vi "Graph Closed.vi"(8 "error in (no error)":errorcluster, 10 "Closed Graph":refnum<class "Message Enqueuer.lvclass">, 11 "Mag Lab Measure Base in":refnum<class "Mag Lab Measure Base.lvclass">) -> (0 "error out":errorcluster, 3 "Mag Lab Measure Base out":refnum<class "Mag Lab Measure Base.lvclass">)   [LabVIEW 2015, in "Mag Lab Measure Base.lvclass"]
uses:
  Mag Lab Measure Base.lvclass
  <vilib>/ActorFramework/Message Enqueuer/Message Enqueuer.lvclass
  Mag Lab Measure Base.lvclass/Mag Lab Measure Base.ctl
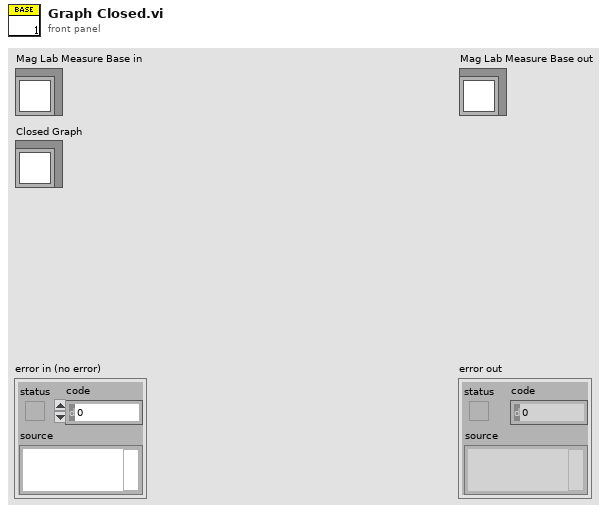
[diagram p1: front panel]
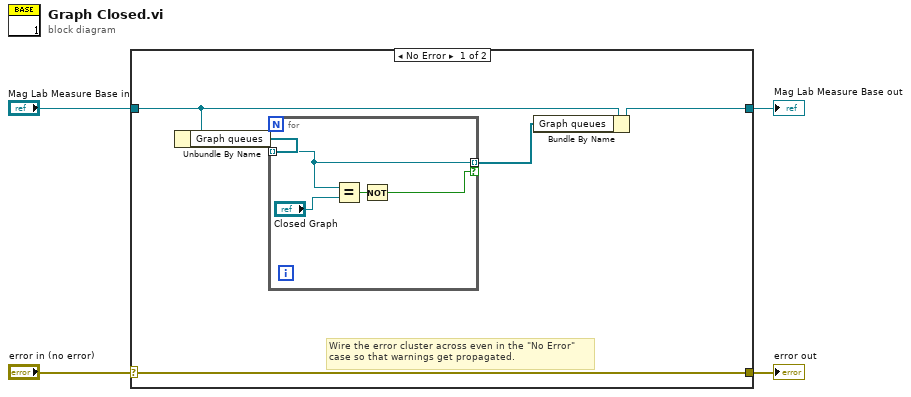
[diagram p0: block diagram]
diagram:
  n1 = case shown="No Error" "error in (no error)" {
    selector: "error in (no error)" -> [w9 w15]
    tunnel: [w9 w15] -> w3
    tunnel: [w6 w14] -> w1
    tunnel: "Mag Lab Measure Base in" -> [w8 w14]
    frame No Error {
      # "Wire the error cluster across even in the \"No Error\"\ncase so that warnings get propagated."
      n2 = Unbundle By Name(w8) -> ("Graph queues"=w7:refnum<class "Message Enqueuer.lvclass">[])
      n3 = for {
        tunnel: w7 -> [w12] mode=indexing
        tunnel: [w12] -> w5 mode=indexing if=w10
        n4 = Equal?(x=w12, y="Closed Graph") -> (x = y?=w11:bool)
        n5 = Not(x=w11) -> (.not. x?=w10:bool)
      }
      n6 = Bundle By Name(cluster=w8, "Graph queues"=w5) -> (w6:refnum<class "Mag Lab Measure Base.lvclass">)
    }
    frame Error {
    }
  }
  "error out" <- w3
  "Mag Lab Measure Base out" <- w1
